vi "CALIBRATE 2016.vi"(0 "flow_slope_IN":dbl=51.35 format="%.2f", 1 "Array in":refnum<k24>[](array[refnum]), 5 "pressure_slope_IN":dbl=23.33 format="%.2f", 7 "Descriptions":string[](array[string]), 9 "string_pot_slope_IN":dbl=1.5 format="%.2f", 11 "error in (no error)":errorcluster, 12 "Sensor Cluster":T1, 14 "Path":path=path "C:/KPRO_2010/Output_files/slopes-cal-record.txt") -> (2 "Array out":refnum<k24>[](array[refnum]), 4 "flow_slope_OUT":dbl=51.35 format="%.2f", 6 "pressure_slope_OUT":dbl=23.33 format="%.2f", 10 "string_pot_slope_OUT":dbl=1.5 format="%.2f", 13 "Sensor Cluster 2":T1, 15 "error out":errorcluster)   [LabVIEW 2016]
uses:
  Waterloo DAQ/controls/MCC DAQ Readings.ctl
  C:/Program Files (x86)/National Instruments/LabVIEW 2016/vi.lib/ULx/ULx_LV.dll
panel:
  in  "exit":bool
  in  "string_pot":bool
  in  "pressure":bool
  in  "flow":bool
  in  "start path":path=path "C:/"
  in  "all":bool
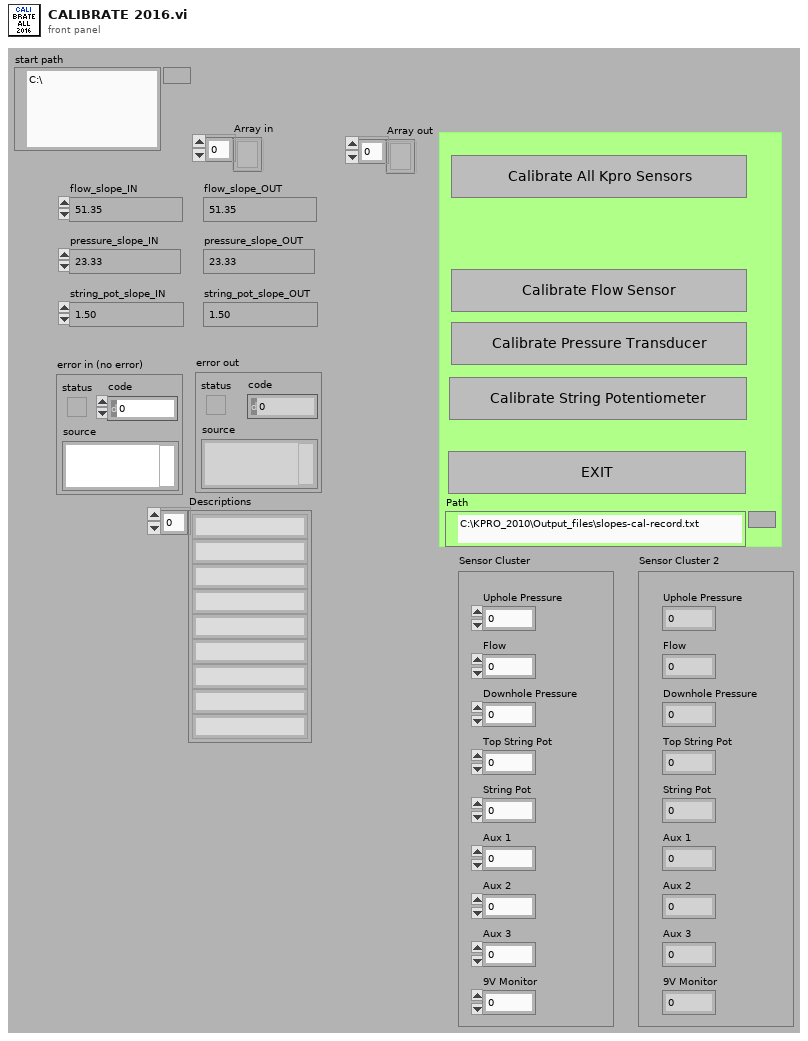
[diagram p1: front panel]
types:
  T1 = typedef "MCC DAQ Readings.ctl" = cluster{"Uphole Pressure":dbl, "Flow":dbl, "Downhole Pressure":dbl, "Top String Pot":dbl, "String Pot":dbl, "Aux 1":dbl, "Aux 2":dbl, "Aux 3":dbl, "9V Monitor":dbl}
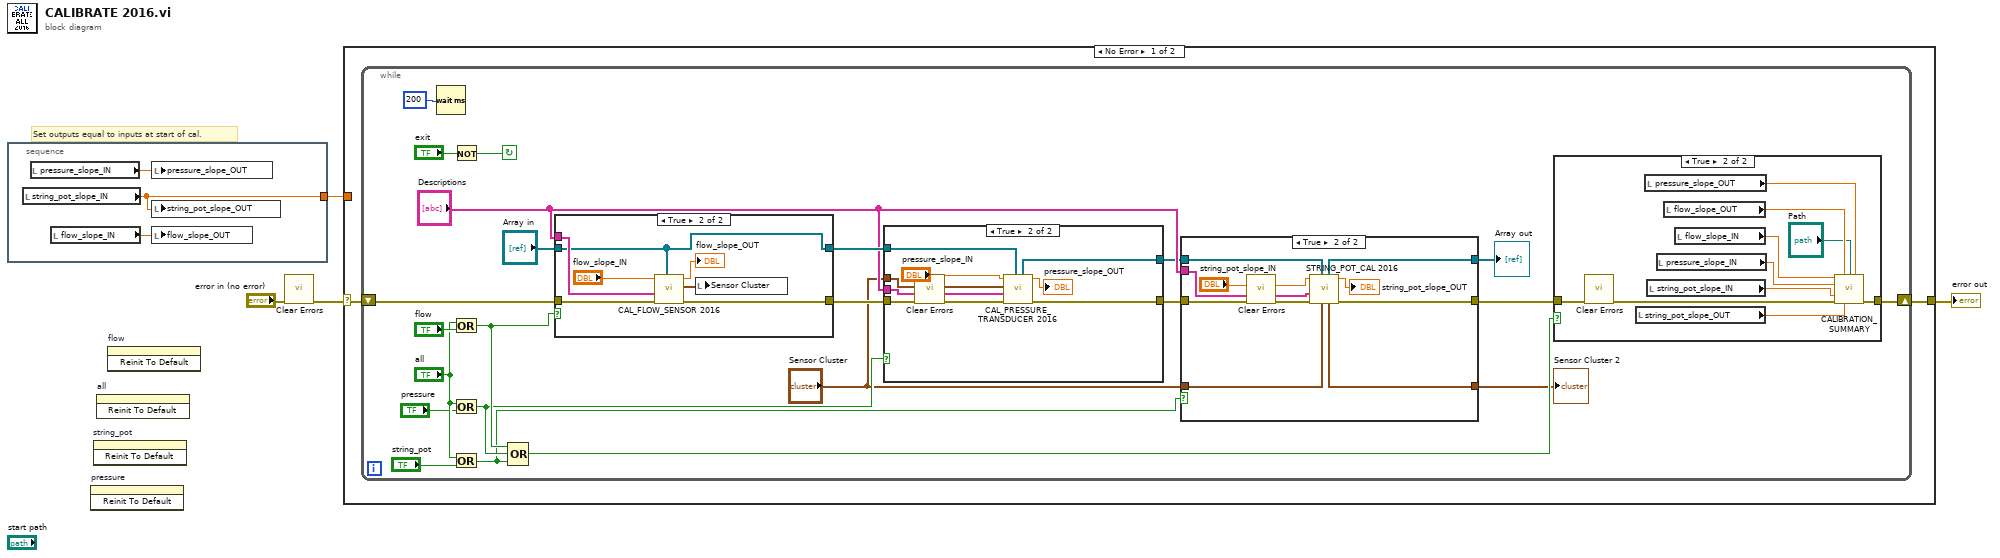
[diagram p0: block diagram]
diagram:
  # "Set outputs equal to inputs at start of cal."
  n1 = stacked-sequence {
    tunnel: [w5] -> w2
    frame #0 {
      n2 = local read "string_pot_slope_IN"() -> (w5:dbl)
      n3 = local read "pressure_slope_IN"() -> (w6:dbl)
      n4 = local read "flow_slope_IN"() -> (w7:dbl)
      n5 = local write "pressure_slope_OUT"(w6) -> ()
      n6 = local write "string_pot_slope_OUT"(w5) -> ()
      n7 = local write "flow_slope_OUT"(w7) -> ()
    }
  }
  n8 = invoke on="pressure" class="Bool" method="Reinit To Default"() -> ()  [unwired: 3 in, 3 out]
  n9 = invoke on="string_pot" class="Bool" method="Reinit To Default"() -> ()  [unwired: 3 in, 3 out]
  n10 = invoke on="all" class="Bool" method="Reinit To Default"() -> ()  [unwired: 3 in, 3 out]
  n11 = invoke on="flow" class="Bool" method="Reinit To Default"() -> ()  [unwired: 3 in, 3 out]
  n12 = call <vilib>:"Clear Errors.vi"("error in (no error)"="error in (no error)") -> ("error out"=w1:errorcluster)  [unwired: 5 in, 1 out]
  n13 = case shown="No Error" w1 {
    selector: w1 -> [w9 w77]
    tunnel: [w8 w77] -> w3
    tunnel: w2 -> [_ _]
    frame No Error {
      n14 = while {
        shift-left: w9 -> [w29]
        shift-right: [w21] -> w8
        stop <- w32 continue-if-true
        n15 = Wait (ms)(milliseconds to wait=u32 200) -> ()  [unwired: 1 out]
        n16 = Not(x="exit") -> (.not. x?=w32:bool)
        n17 = Or(x="all", y="flow") -> (x .or. y?=w20:bool)
        n18 = Or(x="all", y="pressure") -> (x .or. y?=w19:bool)
        n19 = Or(x="all", y="string_pot") -> (x .or. y?=w18:bool)
        n20 = Compound Arithmetic op=OR(w20, w19, w18) -> (w17:bool)
        n21 = case shown="True" w20 {
          tunnel: w29 -> [w69 w76]
          tunnel: [w69 w75] -> w26
          tunnel: "Descriptions" -> [_ w72]
          tunnel: "Array in" -> [w68 w71]
          tunnel: [w68 w71] -> w15
          frame False {
          }
          frame True {
            n22 = call "CAL_FLOW_SENSOR 2016.vi"("Array in"=w71, "error in (no error)"=w76, "Descriptions"=w72, "flow_slope_IN"="flow_slope_IN") -> ("error out"=w75:errorcluster, "Sensor Cluster"=w70:T1, "flow_slope\nmL/min"=→"flow_slope_OUT":dbl)  [unwired: 4 in, 1 out]
            n23 = local write "Sensor Cluster"(w70) -> ()
          }
        }
        n24 = case shown="True" w19 {
          tunnel: [w58 w66] -> w27
          tunnel: w26 -> [w58 w67]
          tunnel: "Sensor Cluster" -> [_ w63]
          tunnel: "Descriptions" -> [_ w62]
          tunnel: w15 -> [w57 w61]
          tunnel: [w57 w60] -> w12
          frame False {
          }
          frame True {
            n25 = call <vilib>:"Clear Errors.vi"("error in (no error)"=w67) -> ("error out"=w59:errorcluster)  [unwired: 5 in, 1 out]
            n26 = call "CAL_PRESSURE_TRANSDUCER 2016.vi"("Array in"=w61, "error in (no error)"=w59, "Descriptions"=w62, "Sensor Cluster"=w63, "pressure_slope_IN"="pressure_slope_IN") -> ("error out"=w66:errorcluster, "pressure_slope_OUT"=→"pressure_slope_OUT":dbl, "Array out"=w60:refnum<k24>[])  [unwired: 3 in, 1 out]
          }
        }
        n27 = case shown="True" w18 {
          tunnel: w27 -> [w46 w50]
          tunnel: [w46 w49] -> w22
          tunnel: "Descriptions" -> [_ w56]
          tunnel: "Sensor Cluster" -> [w45 w55]
          tunnel: w12 -> [w44 w54]
          tunnel: [w44 w53] -> w11
          tunnel: [w45 w48] -> w10
          frame False {
          }
          frame True {
            n28 = call <vilib>:"Clear Errors.vi"("error in (no error)"=w50) -> ("error out"=w47:errorcluster)  [unwired: 5 in, 1 out]
            n29 = call "STRING_POT_CAL 2016.vi"("Sensor Cluster"=w55, "Array in"=w54, "error in (no error)"=w47, "Descriptions"=w56, "string_pot_slope_IN"="string_pot_slope_IN") -> ("error out"=w49:errorcluster, "string_pot_slope_OUT"=→"string_pot_slope_OUT":dbl, "Sensor Cluster 2"=w48:T1, "Array out"=w53:refnum<k24>[])  [unwired: 3 in]
          }
        }
        "Array out" <- w11
        "Sensor Cluster 2" <- w10
        n30 = case shown="True" w17 {
          tunnel: w22 -> [w33 w43]
          tunnel: [w33 w42] -> w21
          frame False {
          }
          frame True {
            n31 = call <vilib>:"Clear Errors.vi"("error in (no error)"=w43) -> ("error out"=w34:errorcluster)  [unwired: 5 in, 1 out]
            n32 = local read "string_pot_slope_OUT"() -> (w36:dbl)
            n33 = local read "pressure_slope_OUT"() -> (w41:dbl)
            n34 = local read "string_pot_slope_IN"() -> (w37:dbl)
            n35 = local read "pressure_slope_IN"() -> (w38:dbl)
            n36 = local read "flow_slope_OUT"() -> (w40:dbl)
            n37 = local read "flow_slope_IN"() -> (w39:dbl)
            n38 = call "CALIBRATION_SUMMARY.vi"("flow_slope_IN"=w39, "flow_slope_OUT"=w40, "Path"="Path", "pressure_slope_OUT"=w41, "pressure_slope_IN"=w38, "string_pot_slope_IN"=w37, "error in (no error)"=w34, "string_pot_slope_OUT"=w36) -> ("error out"=w42:errorcluster)  [unwired: 7 in]
          }
        }
      }
    }
    frame Error {
    }
  }
  "error out" <- w3
